vi "Display Console.vi"(8 "Error In":errorcluster) -> (0 "Error Out":errorcluster)   [LabVIEW 2017]
uses:
  Communication/Reference Action.ctl
panel:
  out "Emergency":bool
  out "Door Open":bool
  in  "Elevator Direction Down":bool
  in  "Elevator Direction Up":bool
  in  "Timing":bool
  in  "Elevator Location":bool
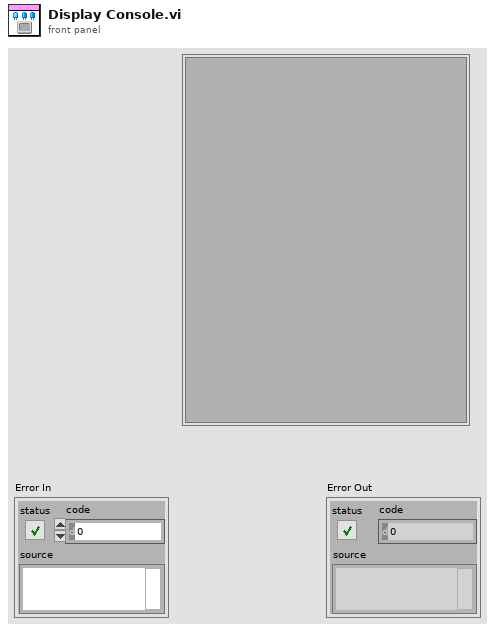
[diagram p1: front panel]
types:
  T1 = typedef "Reference Action.ctl" = enum16{"Set", "Get"}
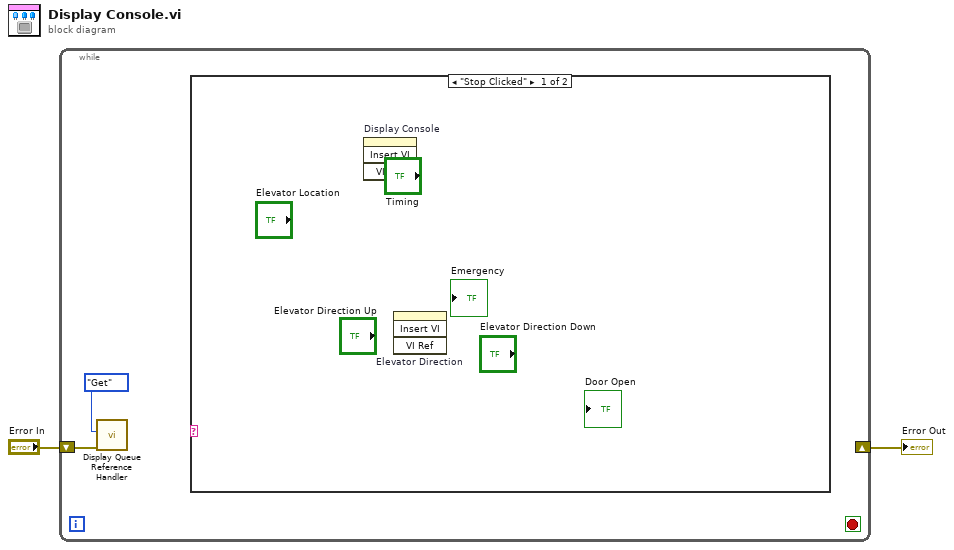
[diagram p0: block diagram]
diagram:
  n1 = while {
    shift-right: [_] -> w1
    shift-left: "Error In" -> [w4]
    stop <- _ stop-if-true
    n2 = call "Display Queue Reference Handler.vi"("Error In"=w4, "Reference Action"=Reference_Action."Get") -> ()  [unwired: 8 in, 2 out]
    n3 = case shown="\"Stop Clicked\"" {
      selector: _ -> [_ _]
      frame "Stop Clicked" {
      }
      frame "True", Default {
      }
    }
  }
  "Error Out" <- w1
  n4 = invoke on="Display Console" class="SubPnl" method="Insert VI"() -> ()  [unwired: 4 in, 4 out]
  n5 = invoke on="Elevator Direction" class="SubPnl" method="Insert VI"() -> ()  [unwired: 4 in, 4 out]
